vi "InitCamGeneral.vi"(8 "error in (no error)":errorcluster) -> (0 "error out":errorcluster)   [LabVIEW 2015, in "ESLSCDLL.lvlib"]
uses:
  ESLSCDLL.lvlib
  Globals.vi
  ESLSCDLL.dll
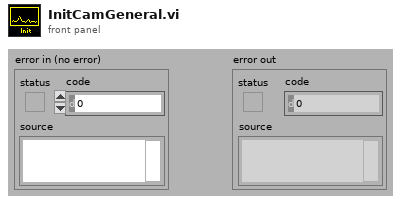
[diagram p1: front panel]
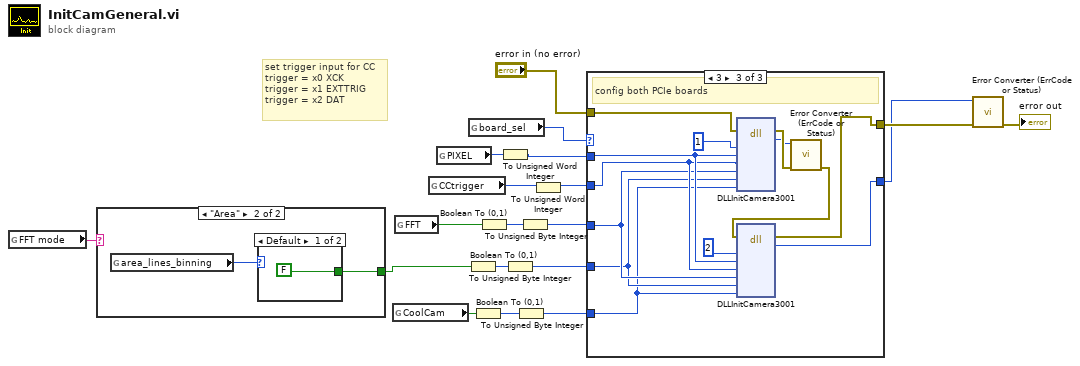
[diagram p0: block diagram]
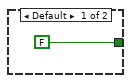
[diagram p2: hidden frame]
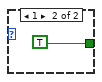
[diagram p3: hidden frame]
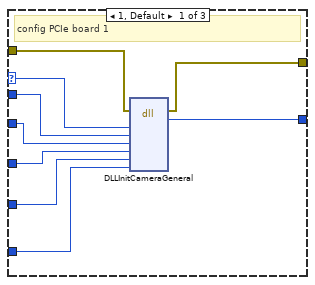
[diagram p4: hidden frame]
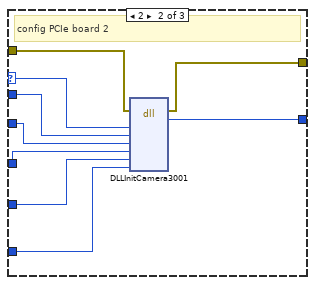
[diagram p5: hidden frame]
diagram:
  # "set trigger input for CC\ntrigger = x0 XCK\ntrigger = x1 EXTTRIG\ntrigger = x2 DAT"
  n1 = global read "Globals.vi" "FFT mode"() -> (w5:string)
  n2 = case shown="\"Area\"" w5 {
    tunnel: [FALSE w21] -> w4
    frame Default {
    }
    frame "Area" {
      n3 = global read "Globals.vi" "area_lines_binning"() -> (w22:u32)
      n4 = case shown="Default" w22 {
        tunnel: [FALSE TRUE] -> w21
        frame Default {
        }
        frame 1 {
        }
      }
    }
  }
  n5 = global read "Globals.vi" "CoolCam"() -> (w6:bool)
  n6 = global read "Globals.vi" "FFT"() -> (w3:bool)
  n7 = global read "Globals.vi" "CCtrigger"() -> (w2:enum16{"XCK", "Ext. Trig.", "DAT"})
  n8 = global read "Globals.vi" "PIXEL"() -> (w8:u32)
  n9 = Boolean To (0,1)(Boolean=w4) -> (0, 1=w18:i16)
  n10 = global read "Globals.vi" "board_sel"() -> (w9:u32)
  n11 = Boolean To (0,1)(Boolean=w6) -> (0, 1=w17:i16)
  n12 = Boolean To (0,1)(Boolean=w3) -> (0, 1=w19:i16)
  n13 = To Unsigned Word Integer(number=w8) -> (unsigned 16bit integer=w7:u16)
  n14 = To Unsigned Byte Integer(number=w18) -> (unsigned 8bit integer=w16:u8)
  n15 = To Unsigned Byte Integer(number=w17) -> (unsigned 8bit integer=w15:u8)
  n16 = To Unsigned Byte Integer(number=w19) -> (unsigned 8bit integer=w14:u8)
  n17 = To Unsigned Word Integer(number=w2) -> (unsigned 16bit integer=w1:u16)
  n18 = case shown="3" w9 {
    selector: w9 -> [w33 w42 _]
    tunnel: w7 -> [w32 w41 w53]
    tunnel: w1 -> [w31 w40 w52]
    tunnel: w14 -> [w30 w39 w51]
    tunnel: w16 -> [w29 w38 w50]
    tunnel: w15 -> [w28 w37 w49]
    tunnel: "error in (no error)" -> [w27 w36 w48]
    tunnel: [w26 w35 w44] -> w11
    tunnel: [w25 w34 w43] -> w10
    frame 1, Default {
      # "config PCIe board 1"
      n19 = dll-call lib="C:/Users/flori/Nextcloud/Dokumente/Stresing/Windows/lv64/board.vis/ESLSCDLL.dll" fn="DLLInitCameraGeneral" ("lwlscdll.dll:DLLWriteLongS0")(error in=w27, "drvno"=w33, "pixel"=w32, "cc_trigger_input"=w31, "IS_FFT"=w30, "IS_AREA"=w29, "IS_COOLED"=w28) -> (error out=w26:errorcluster, "es_status_codes"=w25:i32)  [unwired: 8 in, 1 out]
    }
    frame 2 {
      # "config PCIe board 2"
      n20 = dll-call lib="C:/Users/flori/Nextcloud/Dokumente/Stresing/Windows/lv64/board.vis/ESLSCDLL.dll" fn="DLLInitCamera3001" ("lwlscdll.dll:DLLWriteLongS0")(error in=w36, "drvno"=w42, "pixel"=w41, "cc_trigger_input"=w40, "IS_FFT"=w39, "IS_AREA"=w38, "IS_COOLED"=w37) -> (error out=w35:errorcluster, "es_status_codes"=w34:i32)  [unwired: 8 in, 1 out]
    }
    frame 3 {
      # "config both PCIe boards"
      n21 = dll-call lib="C:/Users/flori/Nextcloud/Dokumente/Stresing/Windows/lv64/board.vis/ESLSCDLL.dll" fn="DLLInitCamera3001" ("lwlscdll.dll:DLLWriteLongS0")(error in=w48, "drvno"=u32 1, "pixel"=w53, "cc_trigger_input"=w52, "IS_FFT"=w51, "IS_AREA"=w50, "IS_COOLED"=w49) -> (error out=w47:errorcluster, "es_status_codes"=w45:i32)  [unwired: 8 in, 1 out]
      n22 = call "Error Converter (ErrCode or Status).vi"("error in (no error)"=w47, "error code"=w45) -> ("error out"=w46:errorcluster)  [unwired: 9 in]
      n23 = dll-call lib="C:/Users/flori/Nextcloud/Dokumente/Stresing/Windows/lv64/board.vis/ESLSCDLL.dll" fn="DLLInitCamera3001" ("lwlscdll.dll:DLLWriteLongS0")(error in=w46, "drvno"=u32 2, "pixel"=w53, "cc_trigger_input"=w52, "IS_FFT"=w51, "IS_AREA"=w50, "IS_COOLED"=w49) -> (error out=w44:errorcluster, "es_status_codes"=w43:i32)  [unwired: 8 in, 1 out]
    }
  }
  n24 = call "Error Converter (ErrCode or Status).vi"("error in (no error)"=w11, "error code"=w10) -> ("error out"=→"error out":errorcluster)  [unwired: 9 in]
